vi "Close.vi"(8 "error in (no error)":errorcluster, 11 "ThermPID in":refnum<class "ThermPID.lvclass">) -> (0 "error out":errorcluster, 3 "ThermPID out":refnum<class "ThermPID.lvclass">)   [LabVIEW 2023, in "ThermPID.lvclass"]
uses:
  ThermPID.lvclass
  ThermPID.lvclass/ThermPID.ctl
  PIDController/PIDController.lvclass
  <vilib>/NI/Modbus Library/API/Master/Modbus Master.lvclass
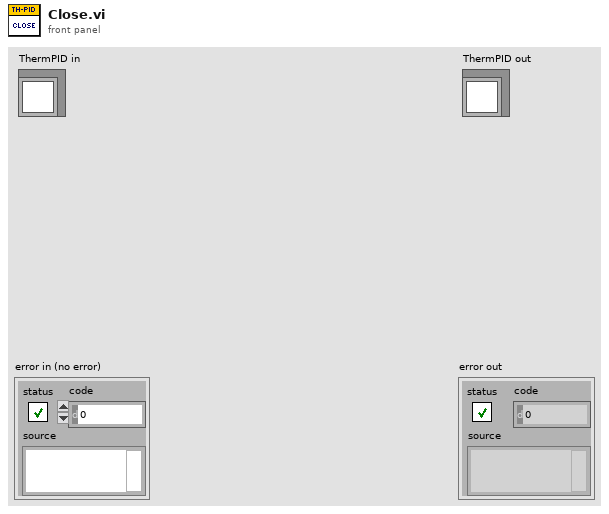
[diagram p1: front panel]
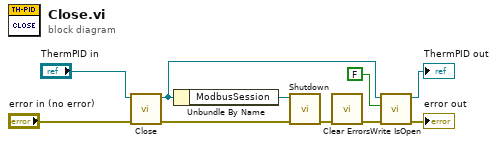
[diagram p0: block diagram]
diagram:
  n1 = call-parent "Close.vi"("error in (no error)"="error in (no error)", "PIDController in"="ThermPID in") -> ("error out"=w7:errorcluster, "PIDController out"=w5:refnum<class "ThermPID.lvclass">)  [unwired: 8 in]
  n2 = Unbundle By Name(w5) -> ("ModbusSession"=w8:refnum<class "Modbus Master.lvclass">)
  n3 = call-dynamic "Shutdown.vi"("error in"=w7, "Modbus master in"=w8) -> ("error out"=w6:errorcluster)  [unwired: 9 in]
  n4 = call <vilib>:"Clear Errors.vi"("error in (no error)"=w6) -> ("error out"=w3:errorcluster)  [unwired: 5 in, 1 out]
  n5 = call-dynamic "Write IsOpen.vi"("error in (no error)"=w3, "IsOpen"=FALSE, "PIDController in"=w5) -> ("error out"=→"error out":errorcluster, "PIDController out"=→"ThermPID out":refnum<class "ThermPID.lvclass">)  [unwired: 7 in]
